vi "PhotonPipelineMetadata_New.vi"(8 "TimeSinceLastPong":i64=9999999999, 9 "SequenceID":i64=-1, 10 "PublishTimestampMicros":i64=-1, 11 "CaptureTimestampMicros":i64=-1) -> (3 "PhotonPipelineMetadata":T1)   [LabVIEW 2019, in "PhotonVisionLib.lvlib"]
doc: "Create new Pipeline MetaData cluster\n\nInputs:\n - CaptureTimestampMicros -- Image capture timestamp, in microseconds\n - PublishTimestampMicros -- NT publish timestamp, in microseconds\n - SequenceID -- Mirror of the heartbeat entry -- monotonically increasing\n - TimeSinceLastPong -- Time from last Time Sync Pong received and the construction of this metadata, in uS\n\nOutputs:\n - PipelineMetaData -- Parsed PipelineMetadata cluster."
uses:
  PhotonVisionLib.lvlib
  TypeDef/PhotonPipelineMetadataType.ctl
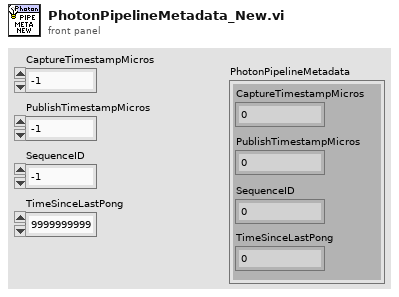
[diagram p1: front panel]
types:
  T1 = typedef "PhotonVisionLib.lvlib/PhotonPipelineMetadataType.ctl" = cluster{"CaptureTimestampMicros":i64, "PublishTimestampMicros":i64, "SequenceID":i64, "TimeSinceLastPong":i64}
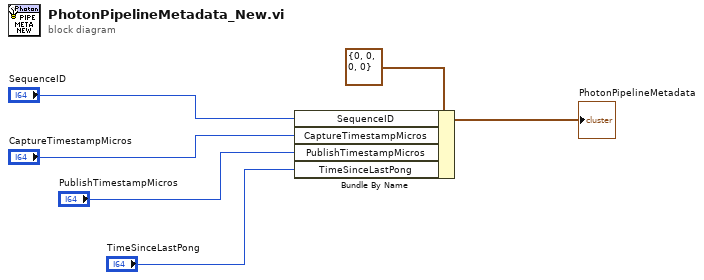
[diagram p0: block diagram]
diagram:
  n1 = Bundle By Name(cluster=T1 {"CaptureTimestampMicros"=0, "PublishTimestampMicros"=0, "SequenceID"=0, "TimeSinceLastPong"=0} ("PhotonPipelineMetadata"), "SequenceID"="SequenceID", "CaptureTimestampMicros"="CaptureTimestampMicros", "PublishTimestampMicros"="PublishTimestampMicros", "TimeSinceLastPong"="TimeSinceLastPong") -> (→"PhotonPipelineMetadata":T1)
